vi "DAQ.DAQmx EventRegistration.vi"(8 "error in (no error)":errorcluster, 10 "DAQmx in":refnum<event-registration>, 11 "Instrument.DAQ in":refnum<class "Instrument.DAQ.lvclass">) -> (0 "error out":errorcluster, 2 "DAQmx out":refnum<event-registration>, 3 "Instrument.DAQ out":refnum<class "Instrument.DAQ.lvclass">)   [LabVIEW 2019, in "Instrument.DAQ.lvclass"]
uses:
  Instrument.DAQ.lvclass
  Instrument.DAQ.lvclass/Instrument.DAQ.ctl
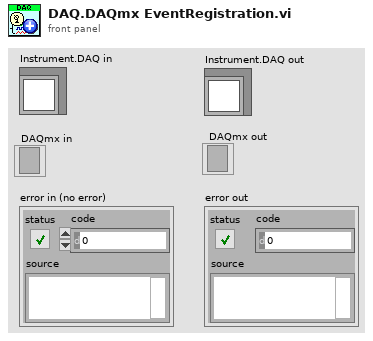
[diagram p1: front panel]
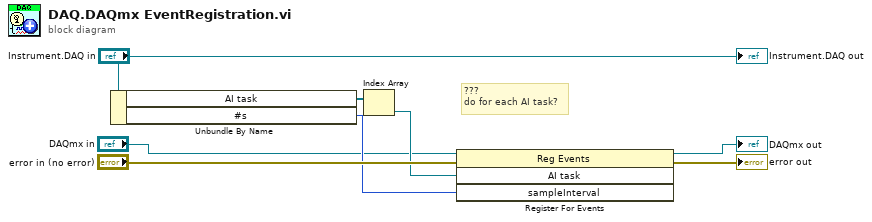
[diagram p0: block diagram]
diagram:
  # "???\ndo for each AI task?"
  n1 = Unbundle By Name("Instrument.DAQ in") -> ("AI task"=w4:refnum<k21>[], "#s"=w3:i32)
  n2 = Index Array(array=w4) -> (element=w2:refnum<k21>)  [unwired: 1 in]
  n3 = register-events(reference="DAQmx in", error in="error in (no error)", w2, w3) -> (reference out=→"DAQmx out":refnum<event-registration>, error out=→"error out":errorcluster)
  "Instrument.DAQ out" <- "Instrument.DAQ in"
